vi "Error Query.vi"(0 "VISA Resource Name":refnum<visa-resource-name>, 11 "error in (no error)":errorcluster) -> (4 "VISA Resource Name Out":refnum<visa-resource-name>, 8 "Error":i32, 10 "Error Message":string, 15 "error out":errorcluster)   [LabVIEW 2018, in "Agilent 34970.lvlib"]
doc: "This VI reads an error from the instrument. It expects to see errors in SCPI format (#,\"error message\"). If an error query is not supported, it returns a warning."
uses:
  Agilent 34970.lvlib
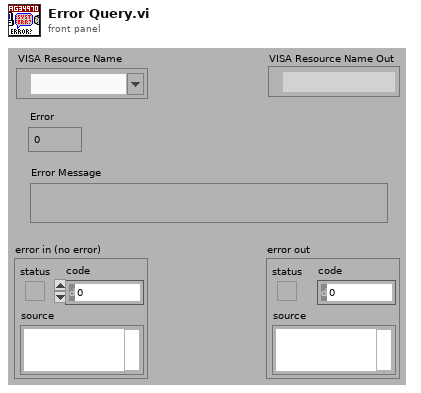
[diagram p1: front panel]
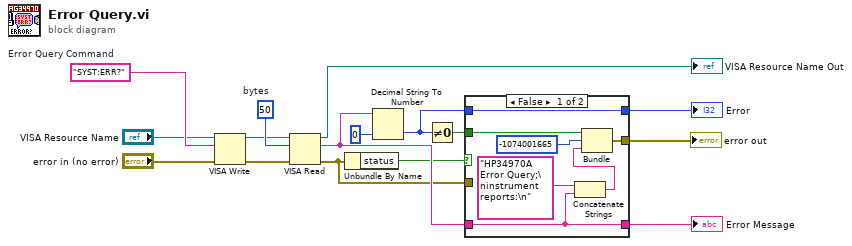
[diagram p0: block diagram]
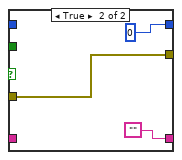
[diagram p2: hidden frame]
diagram:
  w9 = u32 50  # bytes
  w4 = "SYST:ERR?"  # Error Query Command
  n1 = VISA Write(VISA resource name="VISA Resource Name", write buffer=w4, error in (no error)="error in (no error)") -> (VISA resource name out=w8:refnum<visa-resource-name>, error out=w10:errorcluster)  [unwired: 1 out]
  n2 = VISA Read(VISA resource name=w8, byte count=w9, error in (no error)=w10) -> (VISA resource name out=→"VISA Resource Name Out":refnum<visa-resource-name>, read buffer=w13:string, error out=w7:errorcluster)  [unwired: 1 out]
  n3 = Unbundle By Name(w7) -> ("status"=w11:bool)
  n4 = Decimal String To Number(string=w13, default (0L)=0) -> (number=w6:i32)  [unwired: 1 in, 1 out]
  n5 = Not Equal To 0?(x=w6) -> (x != 0?=w12:bool)
  n6 = case shown="False" w11 {
    tunnel: w13 -> [w21 _]
    tunnel: w7 -> [_ w26]
    tunnel: [w19 w26] -> w3
    tunnel: [w21 ""] -> w16
    tunnel: [w18 0] -> w15
    tunnel: w6 -> [w18 _]
    tunnel: w12 -> [w17 _]
    frame False {
      n7 = Concatenate Strings("HP34970A Error Query;\ninstrument reports:\n", w21) -> (w20:string)
      n8 = Bundle(w17, -1074001665, w20) -> (w19:errorcluster)  [unwired: 1 in]
    }
    frame True {
    }
  }
  "Error Message" <- w16
  "Error" <- w15
  "error out" <- w3
